vi "Acquire.vi"(8 "error in (no error)":errorcluster, 11 "SignalWithAlarm in":refnum<class "SignalWithAlarm.lvclass">) -> (0 "error out":errorcluster, 2 "Data":dbl, 3 "SignalWithAlarm out":refnum<class "SignalWithAlarm.lvclass">)   [LabVIEW 2016, in "SignalWithAlarm.lvclass"]
uses:
  SignalWithAlarm.lvclass
  ScalarSignal Class/ScalarSignal.lvclass
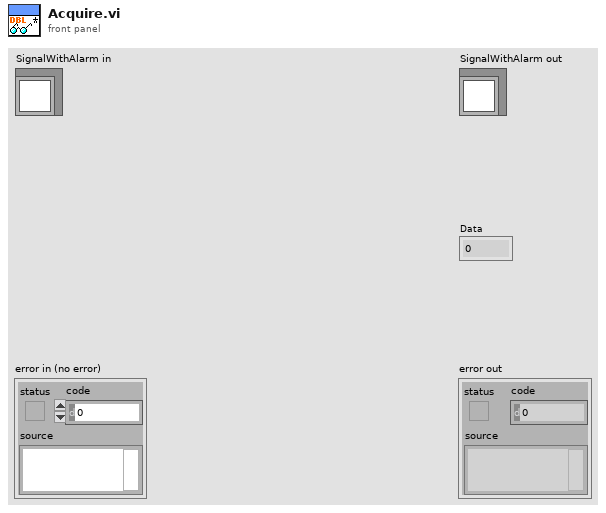
[diagram p1: front panel]
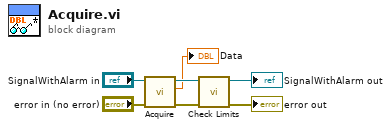
[diagram p0: block diagram]
diagram:
  n1 = call-parent "Acquire.vi"("error in (no error)"="error in (no error)", "ScalarSignal in"="SignalWithAlarm in") -> ("error out"=w3:errorcluster, "Data"=→"Data":dbl, "ScalarSignal out"=w5:refnum<class "SignalWithAlarm.lvclass">)  [unwired: 7 in]
  n2 = call "Check Limits.vi"("error in (no error)"=w3, "SignalWithAlarm in"=w5) -> ("error out"=→"error out":errorcluster, "SignalWithAlarm out"=→"SignalWithAlarm out":refnum<class "SignalWithAlarm.lvclass">)  [unwired: 8 in]
